vi "PID Parameters FG.vi"(7 "Action":T2, 8 "error in (no error)":errorcluster, 10 "Parameters":T3, 11 "Node Ptr":T1 format="%.0x") -> (0 "error out":errorcluster, 2 "Parameters":T3, 3 "Item Ref out":T1=18446744073709551615 format="%.0x")   [LabVIEW 2019, in "Control Addon System Explorer.lvlib"]
uses:
  <vilib>/NI VeriStand/Custom Device API/Custom Device Item Ref.ctl
  Shared/Types/PID Parameters.ctl
  Types/Action.ctl
  Shared/Constants.vi
  <vilib>/NI VeriStand/Custom Device API/Get Item Property (Boolean).vi
  <vilib>/NI VeriStand/Custom Device API/Get Item Property (String).vi
  <vilib>/NI VeriStand/Custom Device API/Set Item Property (Boolean).vi
  <vilib>/NI VeriStand/Custom Device API/Set Item Property (String).vi
  Control Addon System Explorer.lvlib
  <vilib>/NI VeriStand/Custom Device API/Custom Device API.lvlib
  Shared/Control Addon Shared.lvlib
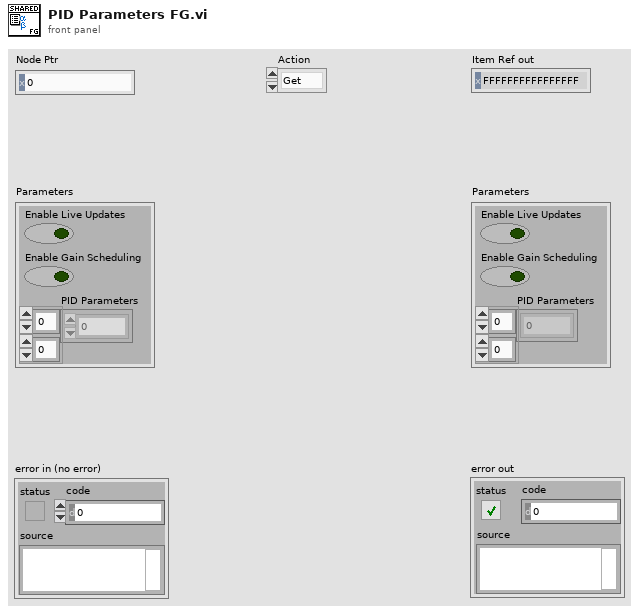
[diagram p1: front panel]
types:
  T1 = typedef "Custom Device API.lvlib/Custom Device Item Ref.ctl" = u64
  T2 = typedef "Control Addon System Explorer.lvlib/Action.ctl" = enum16{"Get", "Set"}
  T3 = typedef "Control Addon Shared.lvlib/PID Parameters.ctl" = cluster{"Enable Live Updates":bool, "Enable Gain Scheduling":bool, "PID Parameters":dbl[][]}
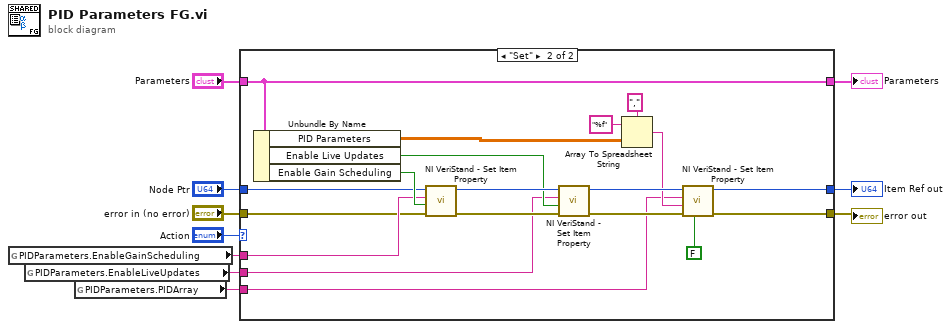
[diagram p0: block diagram]
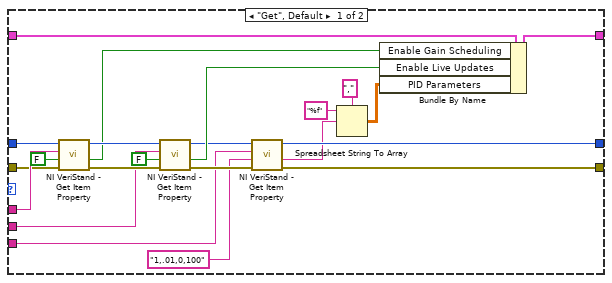
[diagram p2: hidden frame]
diagram:
  n1 = global read "Constants.vi" "PIDParameters.EnableGainScheduling"() -> (w3:string)
  n2 = global read "Constants.vi" "PIDParameters.EnableLiveUpdates"() -> (w2:string)
  n3 = global read "Constants.vi" "PIDParameters.PIDArray"() -> (w1:string)
  n4 = case shown="\"Set\"" "Action" {
    tunnel: "Node Ptr" -> [w25 w43]
    tunnel: "error in (no error)" -> [w26 w44]
    tunnel: "Parameters" -> [w32 w47]
    tunnel: [w31 w47] -> w6
    tunnel: [w19 w41] -> w4
    tunnel: [w21 w39] -> w5
    tunnel: w3 -> [w28 w46]
    tunnel: w2 -> [w27 w45]
    tunnel: w1 -> [w18 w34]
    frame "Get", Default {
      n5 = call-poly <vilib>:"NI VeriStand - Get Item Property.vi"("error in (no error)"=w26, "Default Value"=FALSE, "Property Name"=w28, "Item Ref in"=w25) -> ("error out"=w30:errorcluster, "Value"=w24:bool, "Item Ref out"=w29:T1)  [unwired: 4 in, 1 out]
      n6 = call-poly <vilib>:"NI VeriStand - Get Item Property.vi"("error in (no error)"=w30, "Default Value"=FALSE, "Property Name"=w27, "Item Ref in"=w29) -> ("error out"=w20:errorcluster, "Value"=w23:bool, "Item Ref out"=w22:T1)  [unwired: 4 in, 1 out]
      n7 = call-poly <vilib>:"NI VeriStand - Get Item Property.vi"("error in (no error)"=w20, "Default Value"="1,.01,0,100", "Property Name"=w18, "Item Ref in"=w22) -> ("error out"=w19:errorcluster, "Value"=w17:string, "Item Ref out"=w21:T1)  [unwired: 4 in, 1 out]
      n8 = Spreadsheet String To Array(delimiter (Tab)=",", format string="%f", spreadsheet string=w17) -> (array=w15:dbl[][])  [unwired: 1 in]
      n9 = Bundle By Name(cluster=w32, "Enable Gain Scheduling"=w24, "Enable Live Updates"=w23, "PID Parameters"=w15) -> (w31:T3)
    }
    frame "Set" {
      n10 = Unbundle By Name(w47) -> ("PID Parameters"=w38:dbl[][], "Enable Live Updates"=w48:bool, "Enable Gain Scheduling"=w49:bool)
      n11 = call-poly <vilib>:"NI VeriStand - Set Item Property.vi"("error in (no error)"=w44, "Value"=w49, "Property Name"=w46, "Item Ref in"=w43) -> ("error out"=w50:errorcluster, "Item Ref out"=w51:T1)  [unwired: 5 in, 1 out]
      n12 = call-poly <vilib>:"NI VeriStand - Set Item Property.vi"("error in (no error)"=w50, "Value"=w48, "Property Name"=w45, "Item Ref in"=w51) -> ("error out"=w42:errorcluster, "Item Ref out"=w40:T1)  [unwired: 5 in, 1 out]
      n13 = Array To Spreadsheet String(delimiter (Tab)=",", array=w38, 3:"%f" ("format string")) -> (spreadsheet string=w36:string)
      n14 = call-poly <vilib>:"NI VeriStand - Set Item Property.vi"("Binary String (T)"=FALSE, "error in (no error)"=w42, "Value"=w36, "Property Name"=w34, "Item Ref in"=w40) -> ("error out"=w41:errorcluster, "Item Ref out"=w39:T1)  [unwired: 4 in, 1 out]
    }
  }
  "Parameters" <- w6
  "Item Ref out" <- w5
  "error out" <- w4
